vi "Wire Indicators.vi"(0 "Diagram in":refnum<vi>, 5 "Indicator Names":string[](array[string]), 7 "Outputs":refnum<vi>[](array[refnum]), 11 "error in (no error)":errorcluster) -> (4 "Diagram out":refnum<vi>, 15 "error out":errorcluster)   [LabVIEW 2015, in "Scripting.lvlib"]
doc: "<B>Outputs</B> is an array of terminals to wire to the input terminals of the indicators selected with <B>Indicator Names</b> on <B>Diagram in</B>."
uses:
  Scripting.lvlib
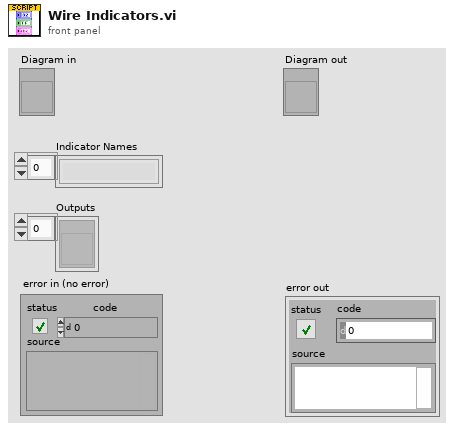
[diagram p1: front panel]
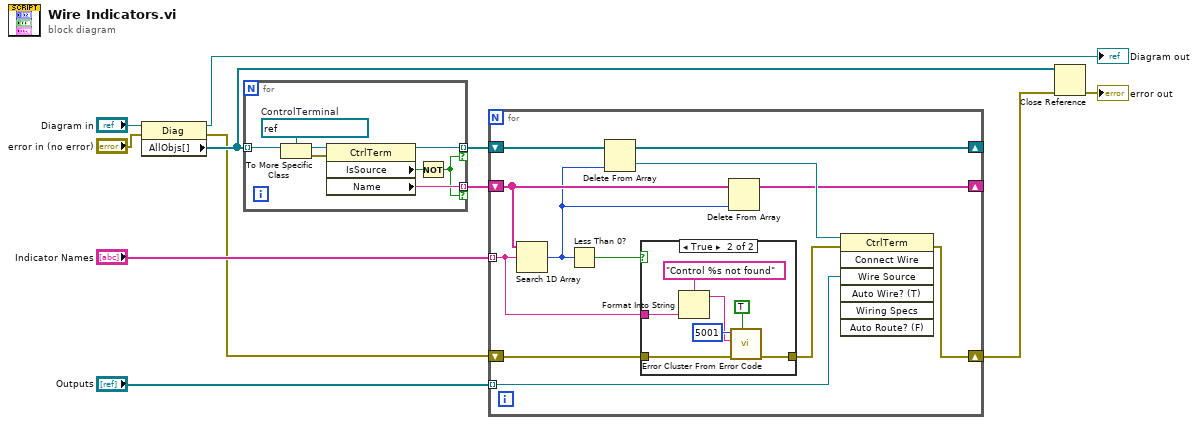
[diagram p0: block diagram]
diagram:
  n1 = property class="Diag"(reference="Diagram in", error in="error in (no error)") -> (reference out=→"Diagram out":refnum<vi>, error out=w2:errorcluster, "AllObjs[]"=w3:refnum<vi>[])
  n2 = for {
    tunnel: w3 -> [w13] mode=indexing
    tunnel: [w14] -> w8 mode=indexing if=w15
    tunnel: [w16] -> w7 mode=indexing if=w15
    w19 = refnum<vi> refnum  # ControlTerminal
    n3 = To More Specific Class(target class=w19, reference=w13) -> (specific class reference=w18:refnum<vi>, error out=w17:errorcluster)  [unwired: 1 in]
    n4 = property class="CtrlTerm"(reference=w18, error in=w17) -> (reference out=w14:refnum<vi>, "IsSource"=w12:bool, "Name"=w16:string)  [unwired: 1 out]
    n5 = Not(x=w12) -> (.not. x?=w15:bool)
  }
  n6 = for {
    tunnel: "Indicator Names" -> [w28] mode=indexing
    shift-right: [w26] -> w1
    shift-left: w2 -> [w29]
    tunnel: "Outputs" -> [w24] mode=indexing
    shift-right: [w21] -> _
    shift-left: w7 -> [w23]
    shift-right: [w20] -> _
    shift-left: w8 -> [w31]
    n7 = Search 1D Array(1D array=w23, element=w28) -> (index of element=w22:i32)  [unwired: 1 in]
    n8 = Less Than 0?(x=w22) -> (x < 0?=w30:bool)
    n9 = Delete From Array(array=w31, index=w22) -> (deleted portion=w27:refnum<vi>, array with subset deleted=w20:refnum<vi>[])  [unwired: 1 in]
    n10 = case shown="True" w30 {
      tunnel: w29 -> [w32 w38]
      tunnel: w28 -> [_ w36]
      tunnel: [w32 w33] -> w25
      frame False {
      }
      frame True {
        n11 = Format Into String(format string="Control %s not found", w36) -> (resulting string=w35:string)  [unwired: 2 in, 1 out]
        n12 = call <vilib>:"Error Cluster From Error Code.vi"("show call chain? (False)"=TRUE, "error in (no error)"=w38, "error message (\"\")"=w35, "error code (0)"=5001) -> ("error out"=w33:errorcluster)  [unwired: 5 in]
      }
    }
    n13 = Delete From Array(array=w23, index=w22) -> (array with subset deleted=w21:string[])  [unwired: 1 in, 1 out]
    n14 = invoke class="CtrlTerm" method="Connect Wire"(reference=w27, error in=w25, "Wire Source"=w24) -> (error out=w26:errorcluster)  [unwired: 4 in, 6 out]
  }
  n15 = Close Reference(reference=w3, error in (no error)=w1) -> (error out=→"error out":errorcluster)
